vi "GrayOutButtonFromPSPVar.vi"(10 "shared variable refnum in":refnum<k21>, 11 "Boolean in":refnum<vi>) -> ()   [LabVIEW 2019]
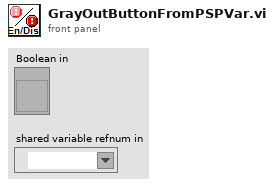
[diagram p1: front panel]
types:
  T1 = enum8{"Enabled", "Disabled", "Disabled and Grayed Out"}
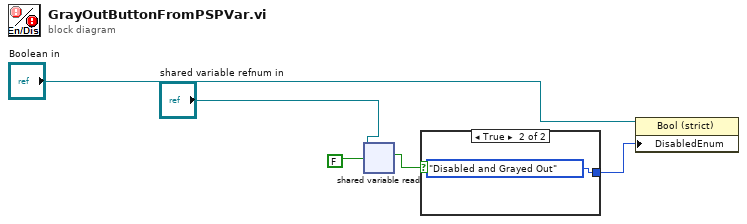
[diagram p0: block diagram]
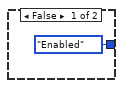
[diagram p2: hidden frame]
diagram:
  n1 = shared-variable-read("shared variable refnum in", FALSE) -> (w3:bool)  [unwired: 1 in, 3 out]
  n2 = case shown="True" w3 {
    tunnel: [T1."Enabled" ("Disabled") T1."Disabled and Grayed Out" ("Disabled")] -> w4
    frame False {
    }
    frame True {
    }
  }
  n3 = property class="Bool (strict)"(reference="Boolean in", "DisabledEnum"=w4) -> ()  [unwired: 1 in, 2 out]
